vi "Initialize.vi"(8 "error in":errorcluster, 11 "Plugin in":refnum<class "MP750510.lvclass">) -> (0 "error out":errorcluster, 3 "Plugin out":refnum<class "MP750510.lvclass">)   [LabVIEW 2025, in "MP750510.lvlib" / "MP750510.lvclass"]
uses:
  MP750510.lvclass
  C:/Program Files/National Instruments/LabVIEW 2025/vi.lib/FlexLogger/SDK/PluginSDK.lvlibp/PEFClasses/SDK/Plugin/Plugin.lvclass
  <vilib>/FlexLogger/SDK/PluginSDK.lvlibp/PEFClasses/SDK/Processing Element/Timing Parameters.ctl
  <vilib>/FlexLogger/SDK/PluginSDK.lvlibp/PEFClasses/SDK/Processing Element/Timing Method.ctl
  <vilib>/FlexLogger/SDK/PluginSDK.lvlibp/PEFClasses/SDK/Setpoint Consumer Channel/Setpoint Consumer Channel.lvclass
  C:/Program Files/National Instruments/LabVIEW 2025/vi.lib/FlexLogger/SDK/PluginSDK.lvlibp/PEFClasses/SDK/Channel/Channel.lvclass
  <vilib>/FlexLogger/SDK/PluginSDK.lvlibp/PEFClasses/SDK/Plugin/ParameterAccess/Write String.vi
  <vilib>/FlexLogger/SDK/PluginSDK.lvlibp/PEFClasses/SDK/Setpoint Consumer Channel/Create Setpoint Consumer Channel.vi
  <vilib>/FlexLogger/SDK/PluginSDK.lvlibp/PEFClasses/SDK/Channel/ParameterAccess/Write DBL.vi
  <vilib>/FlexLogger/SDK/PluginSDK.lvlibp/PEFClasses/SDK/Channel/ParameterAccess/Write Enum.vi
  <vilib>/FlexLogger/SDK/PluginSDK.lvlibp/PEFClasses/SDK/Plugin/Plugin.lvclass
  <vilib>/FlexLogger/SDK/PluginSDK.lvlibp/PEFClasses/SDK/Processing Element/Processing Element.lvclass
  <vilib>/FlexLogger/SDK/PluginSDK.lvlibp/PEFClasses/SDK/Channel/Channel.lvclass
  <vilib>/FlexLogger/SDK/PluginSDK.lvlibp
  <vilib>/FlexLogger/SDK/PluginSDK.lvlibp/PEFClasses/SDK/Parameters/Parameters.lvclass
  C:/Program Files/National Instruments/LabVIEW 2025/vi.lib/FlexLogger/SDK/PluginSDK.lvlibp/PEFClasses/SDK/Consumer Channel/Consumer Channel.lvclass
  C:/Program Files/National Instruments/LabVIEW 2025/vi.lib/FlexLogger/SDK/PluginSDK.lvlibp/PEFClasses/SDK/Setpoint Consumer Channel/Setpoint Consumer Channel.lvclass
  C:/Program Files/National Instruments/LabVIEW 2025/vi.lib/FlexLogger/SDK/PluginSDK.lvlibp/PEFClasses/SDK/Processing Element/Processing Element.lvclass
  C:/Users/Steve/Documents/Git/MP750510_Plugin/FlexLogger/MP750510/MP750510.lvclass
panel:
  out "Array":string[](array[string])
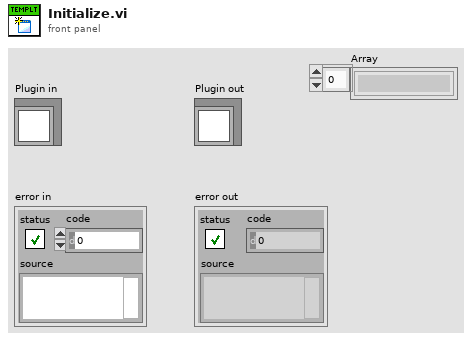
[diagram p1: front panel]
types:
  T1 = typedef "PluginSDK.lvlibp/Processing Element.lvclass/Timing Parameters.ctl" = cluster{"Timing Method":T2, "Timing Period (ms)":i32}
  T2 = typedef "PluginSDK.lvlibp/Processing Element.lvclass/Timing Method.ctl" = enum16{"Periodic", "Immediate", "On Data Ready", "Triggered"}
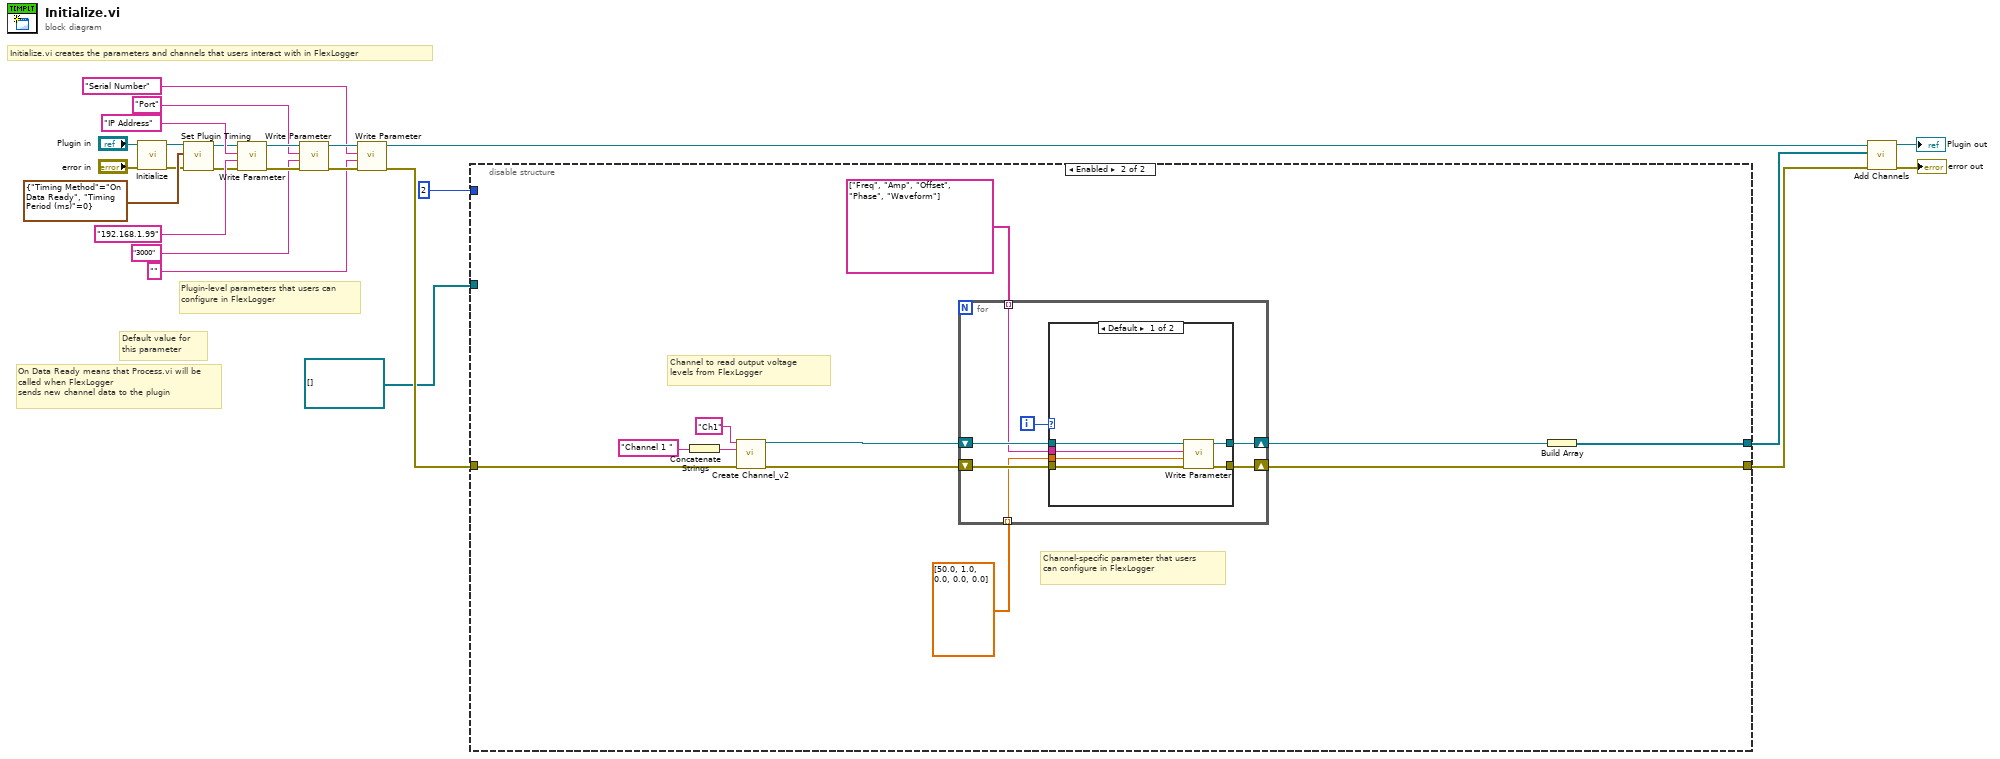
[diagram p0: block diagram]
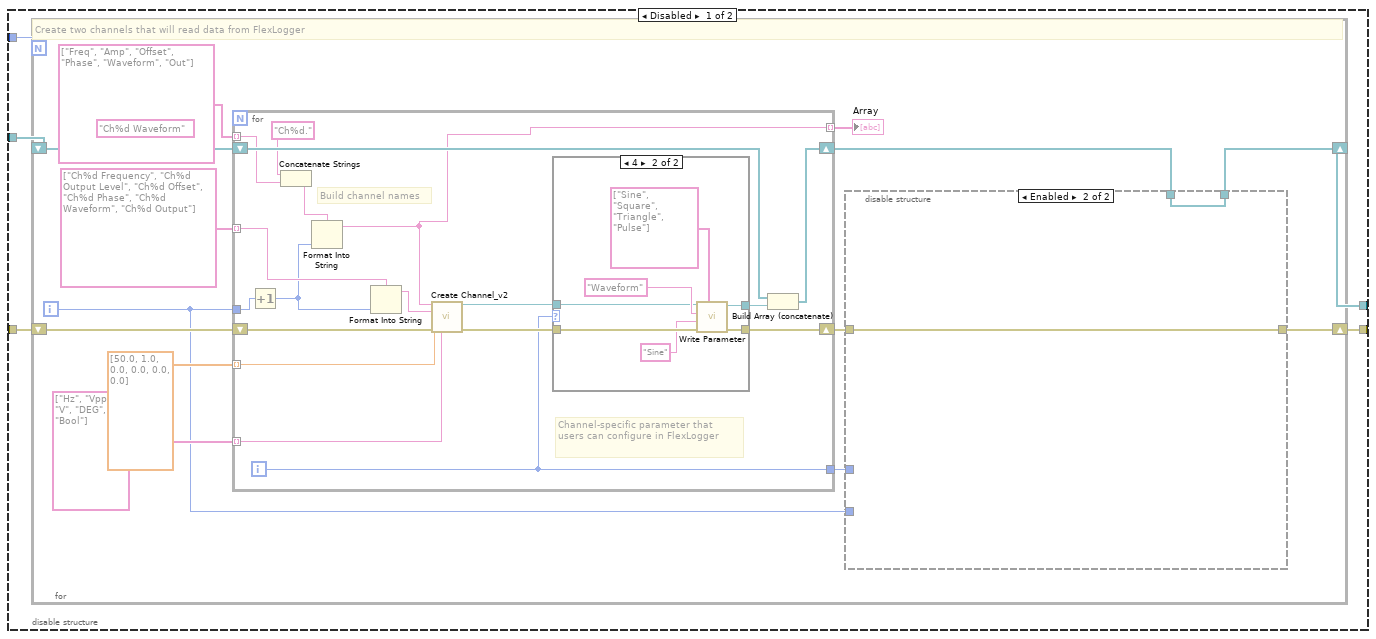
[diagram p2: hidden frame]
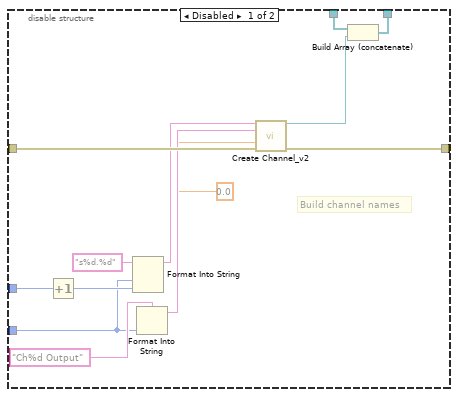
[diagram p3: hidden frame]
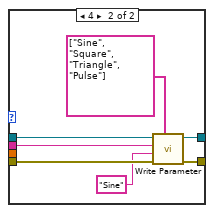
[diagram p5: hidden frame]
diagram:
  # "Default value for this parameter"
  # "Plugin-level parameters that users can configure in FlexLogger"
  # "On Data Ready means that Process.vi will be called when FlexLogger \nsends new channel data to the plugin"
  # "Initialize.vi creates the parameters and channels that users interact with in FlexLogger"
  n1 = call-parent "Initialize.vi"("error in (no error)"="error in", "Plugin in"="Plugin in") -> ("error out"=w14:errorcluster, "Plugin out"=w13:refnum<class "MP750510.lvclass">)  [unwired: 8 in]
  n2 = call <vilib>:"Set Plugin Timing.vi"("error in (no error)"=w14, "Timing Parameters"=T1 {"Timing Method"=enum."On Data Ready", "Timing Period (ms)"=0}, "Plugin in"=w13) -> ("error out"=w11:errorcluster, "Plugin out"=w12:refnum<class "MP750510.lvclass">)  [unwired: 7 in]
  n3 = call-poly <vilib>:"Write Parameter.vi"("error in (no error)"=w11, "Value"="192.168.1.99", "Name"="IP Address", "Plugin in"=w12) -> ("error out"=w17:errorcluster, "Plugin out"=w16:refnum<class "MP750510.lvclass">)  [unwired: 6 in]
  n4 = call-poly <vilib>:"Write Parameter.vi"("error in (no error)"=w17, "Value"="3000", "Name"="Port", "Plugin in"=w16) -> ("error out"=w8:errorcluster, "Plugin out"=w6:refnum<class "MP750510.lvclass">)  [unwired: 6 in]
  n5 = call-poly <vilib>:"Write Parameter.vi"("error in (no error)"=w8, "Value"="", "Name"="Serial Number", "Plugin in"=w6) -> ("error out"=w7:errorcluster, "Plugin out"=w5:refnum<class "MP750510.lvclass">)  [unwired: 6 in]
  n6 = disable-structure shown="Enabled" {
    disable-tunnel: 2 -> [w30 _]
    disable-tunnel: [w29 w89] -> w20
    disable-tunnel: w7 -> [w28 w90]
    disable-tunnel: refnum<class "Setpoint Consumer Channel.lvclass">[] [] -> [w27 _]
    disable-tunnel: [w26 w88] -> w1
    frame Disabled {
      n7 = for {
        N: w30 -> [_]
        shift-right: [w33] -> w29
        shift-left: w28 -> [w43]
        shift-right: [w36] -> w26
        shift-left: w27 -> [w37]
        i -> [w34]
        (unwired) "Ch%d Waveform" ("format string")
        # "Create two channels that will read data from FlexLogger"
        n8 = for {
          tunnel: w34 -> [w63]
          tunnel: string[] ["Ch%d Frequency", "Ch%d Output Level", "Ch%d Offset", "Ch%d Phase", "Ch%d Waveform", "Ch%d Output"] -> [w71] mode=indexing
          shift-right: [w75] -> w39
          shift-left: w43 -> [w73]
          tunnel: string[] ["Hz", "Vpp", "V", "DEG", "", "Bool"] -> [w70] mode=indexing
          tunnel: dbl[] [50.0, 1.0, 0.0, 0.0, 0.0, 0.0] -> [w69] mode=indexing
          shift-right: [w67] -> w38
          shift-left: w37 -> [w66]
          tunnel: [w65] -> w35
          tunnel: string[] ["Freq", "Amp", "Offset", "Phase", "Waveform", "Out"] -> [w64] mode=indexing
          tunnel: [w59] -> w31 mode=indexing
          i -> [w65]
          # "Build channel names"
          # "Channel-specific parameter that users can configure in FlexLogger"
          n9 = Increment(x=w63) -> (x+1=w62:i32)
          n10 = Concatenate Strings("Ch%d." ("format string"), w64) -> (w60:string)
          n11 = Format Into String(format string=w60, w62) -> (resulting string=w59:string)  [unwired: 2 in, 1 out]
          n12 = Format Into String(format string=w71, w62) -> (resulting string=w76:string)  [unwired: 2 in, 1 out]
          n13 = call-poly <vilib>:"Create Channel_v2.vi"("Unique Channel Identifier"=w59, "Default Channel Name"=w76, "Default Value"=w69, "error in (no error)"=w73, "Unit"=w70) -> ("Setpoint Consumer Channel"=w74:refnum<class "Setpoint Consumer Channel.lvclass">, "error out"=w72:errorcluster)  [unwired: 9 in]
          n14 = case shown="4" w65 {
            tunnel: [w77 w84] -> w75
            tunnel: w74 -> [w78 w83]
            tunnel: [w78 w82] -> w68
            tunnel: w72 -> [w77 w81]
            frame Default {
            }
            frame 4 {
              n15 = call-poly <vilib>:"Write Parameter.vi"("Possible Values"=string[] ["Sine", "Square", "Triangle", "Pulse"], "error in (no error)"=w81, "Current Value"="Sine" ("format string"), "Name"="Waveform", "Channel in"=w83) -> ("error out"=w84:errorcluster, "Channel out"=w82:refnum<class "Setpoint Consumer Channel.lvclass">)  [unwired: 5 in]
            }
          }
          n16 = Build Array (concatenate)(w66, w68) -> (w67:refnum<class "Setpoint Consumer Channel.lvclass">[])
        }
        "Array" <- w31
        n17 = disable-structure shown="Enabled" {
          disable-tunnel: w39 -> [w56 w58]
          disable-tunnel: w38 -> [w55 w57]
          disable-tunnel: [w54 w57] -> w36
          disable-tunnel: w35 -> [w53 _]
          disable-tunnel: w34 -> [w48 _]
          disable-tunnel: [w45 w58] -> w33
          frame Disabled {
            # "Build channel names"
            n18 = Increment(x=w53) -> (x+1=w51:i32)
            n19 = Format Into String(format string="s%d.%d", w48, w51) -> (resulting string=w50:string)  [unwired: 2 in, 1 out]
            n20 = Format Into String(format string="Ch%d Output", w48) -> (resulting string=w47:string)  [unwired: 2 in, 1 out]
            n21 = call-poly <vilib>:"Create Channel_v2.vi"("Unique Channel Identifier"=w50, "Default Channel Name"=w47, "Default Value"=0.0, "error in (no error)"=w56) -> ("Setpoint Consumer Channel"=w44:refnum<class "Setpoint Consumer Channel.lvclass">, "error out"=w45:errorcluster)  [unwired: 10 in]
            n22 = Build Array (concatenate)(w55, w44) -> (w54:refnum<class "Setpoint Consumer Channel.lvclass">[])
          }
          frame Enabled {
          }
        }
      }
    }
    frame Enabled {
      # "Channel to read output voltage levels from FlexLogger"
      # "Channel-specific parameter that users can configure in FlexLogger"
      n23 = Concatenate Strings("Channel 1 " ("format string")) -> (w91:string)
      n24 = call-poly <vilib>:"Create Channel_v2.vi"("Unique Channel Identifier"="Ch1" ("Source"), "Default Channel Name"=w91, "error in (no error)"=w90) -> ("Setpoint Consumer Channel"=w94:refnum<class "Setpoint Consumer Channel.lvclass">, "error out"=w95:errorcluster)  [unwired: 11 in]
      n25 = for {
        shift-right: [w102] -> w89
        shift-left: w95 -> [w100]
        shift-right: [w103] -> w96
        shift-left: w94 -> [w101]
        tunnel: string[] ["Freq", "Amp", "Offset", "Phase", "Waveform"] -> [w98] mode=indexing
        tunnel: dbl[] [50.0, 1.0, 0.0, 0.0, 0.0] -> [w97] mode=indexing
        i -> [w99]
        n26 = case shown="Default" w99 {
          tunnel: [w106 w116] -> w102
          tunnel: w101 -> [w109 w115]
          tunnel: [w105 w114] -> w103
          tunnel: w100 -> [w108 w113]
          tunnel: w98 -> [w107 w110]
          tunnel: w97 -> [w104 _]
          frame Default {
            n27 = call-poly <vilib>:"Write Parameter.vi"("error in (no error)"=w108, "Value"=w104, "Name"=w107, "Channel in"=w109) -> ("error out"=w106:errorcluster, "Channel out"=w105:refnum<class "Setpoint Consumer Channel.lvclass">)  [unwired: 6 in]
          }
          frame 4 {
            n28 = call-poly <vilib>:"Write Parameter.vi"("Possible Values"=string[] ["Sine", "Square", "Triangle", "Pulse"], "error in (no error)"=w113, "Current Value"="Sine" ("format string"), "Name"=w110, "Channel in"=w115) -> ("error out"=w116:errorcluster, "Channel out"=w114:refnum<class "Setpoint Consumer Channel.lvclass">)  [unwired: 5 in]
          }
        }
      }
      n29 = Build Array(w96) -> (w88:refnum<class "Setpoint Consumer Channel.lvclass">[])
    }
  }
  n30 = call <vilib>:"Add Channels.vi"("error in (no error)"=w20, "Channels"=w1, "Plugin in"=w5) -> ("error out"=→"error out":errorcluster, "Plugin out"=→"Plugin out":refnum<class "MP750510.lvclass">)  [unwired: 7 in]
